vi "New Blob.vi"(10 "rect":T1) -> (3 "Blob out":refnum<class "Blob.lvclass">)   [LabVIEW 2023, in "Blob.lvclass"]
doc: "Create a new Blob object."
uses:
  Blob.lvclass
  <vilib>/Utility/miscctls.llb/LVRectTypeDef.ctl
  Blob.lvclass/Blob.ctl
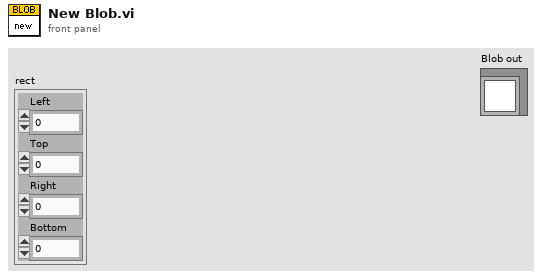
[diagram p1: front panel]
types:
  T1 = typedef "LVRectTypeDef.ctl" = cluster{"Left":i16, "Top":i16, "Right":i16, "Bottom":i16}
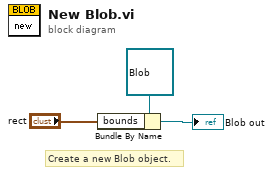
[diagram p0: block diagram]
diagram:
  # "Create a new Blob object."
  n1 = Bundle By Name(cluster=refnum<class "Blob.lvclass"> refnum ("Blob out"), "bounds"="rect") -> (→"Blob out":refnum<class "Blob.lvclass">)
